vi "ControlSystemTemplate.vi"() -> ()   [LabVIEW 2012]
uses:
  SingleControls/TypeDef_LoopStages.ctl
  GlobalVariables_DIALMain.vi
  <vilib>/Utility/miscctls.llb/LVRectTypeDef.ctl
  <vilib>/Utility/miscctls.llb/LVPointTypeDef.ctl
panel:
  out "Commands Executed":i32
  in  "Reset Plot Bounds":bool
  out "Local Loop Stage":T1=enum."Exit"
  out "Total Errors":i32
  out "Permission Level":T2(ring)
  out "Local Queue Response":string="Exit Idle Loop"
  in  "Replot":bool
  in  "User Comment":bool
  in  "Update Permissions":bool
  in  "Software Testing":bool
  in  "Commanded Abort":bool
  out "Waiting Commands":i32
  out "Local Queue Element":string="Exit"
  in  "Local Abort":bool=TRUE
  # "Place Hidden Variables Here"
  # "Place Controls Here"
  # "Panel width is 954\nPanel height is 700 as child\nPanel height is 783 as stand alone"
  # "Place Queue Housekeeping Here"
  # "Place Global Buttons Here"
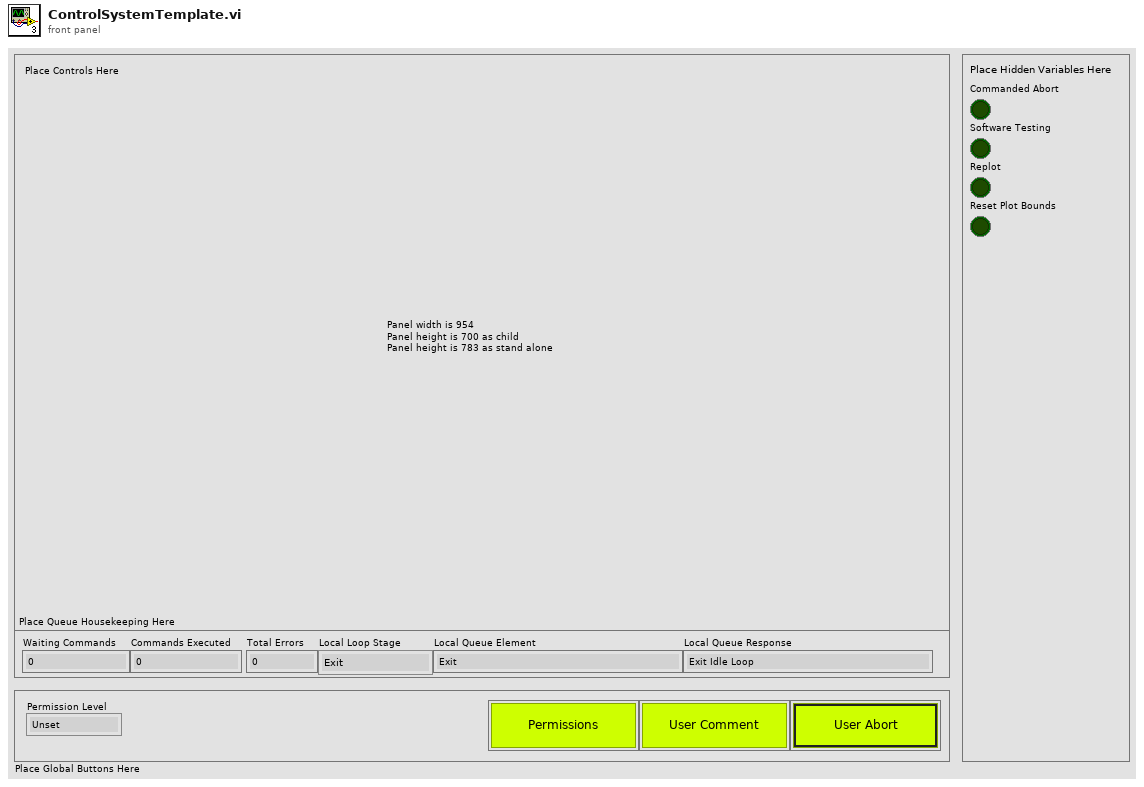
[diagram p1: front panel]
types:
  T1 = typedef "TypeDef_LoopStages.ctl" = enum16{"Configure", "Initialize", "Idle", "Error Handler", "Commanded Exit", "Exit"}
  T2 = enum16{"Unset", "Operator", "Administrator", "Full"}
  T3 = typedef "LVPointTypeDef.ctl" = cluster{"Horizontal":i16, "Vertical":i16}
  T4 = typedef "LVRectTypeDef.ctl" = cluster{"Left":i16, "Top":i16, "Right":i16, "Bottom":i16}
  T5 = enum16{"Always On", "Always Off", "Off While Running"}
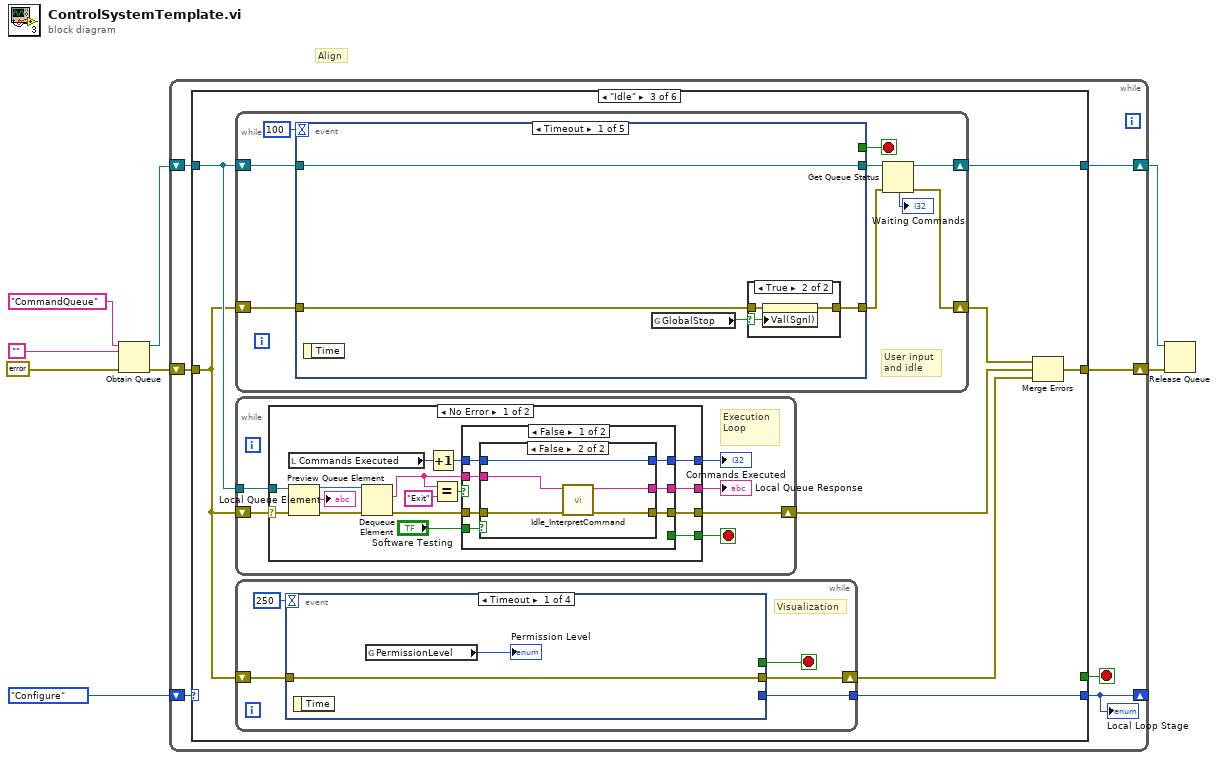
[diagram p0: block diagram]
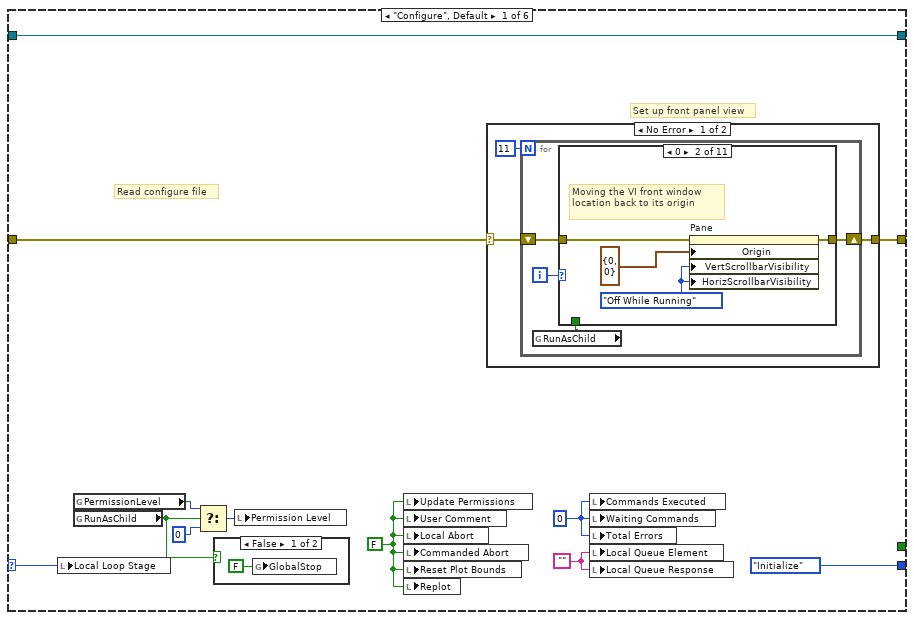
[diagram p2: hidden frame]
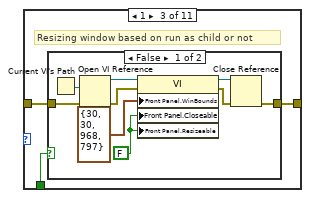
[diagram p5: hidden frame]
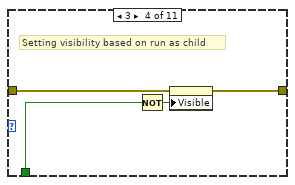
[diagram p7: hidden frame]
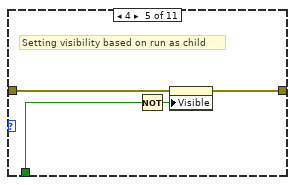
[diagram p8: hidden frame]
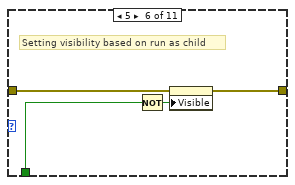
[diagram p9: hidden frame]
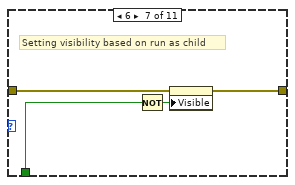
[diagram p10: hidden frame]
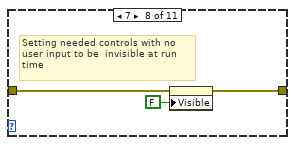
[diagram p11: hidden frame]
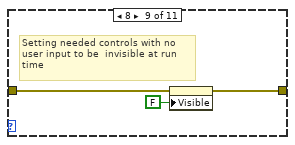
[diagram p12: hidden frame]
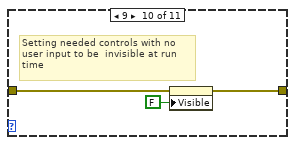
[diagram p13: hidden frame]
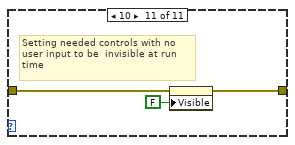
[diagram p14: hidden frame]
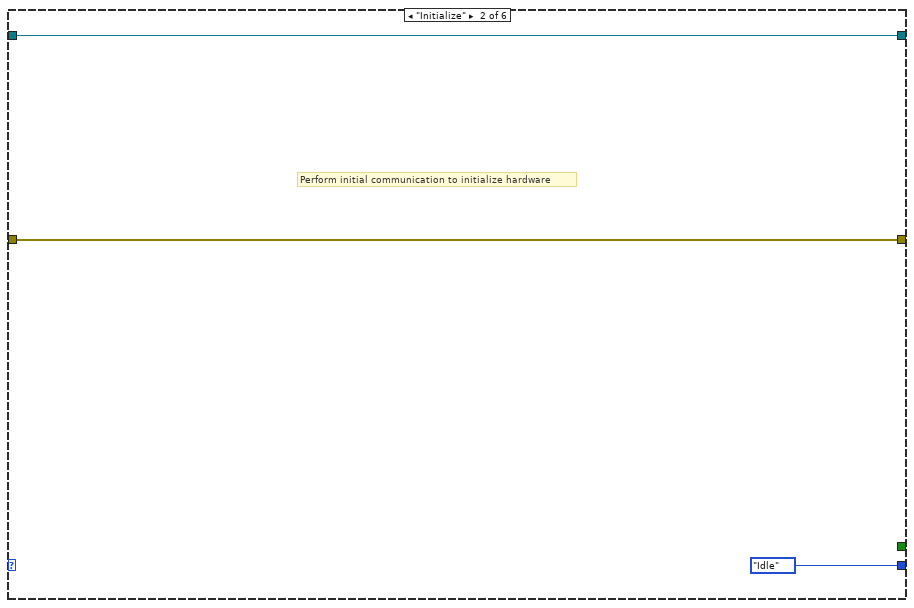
[diagram p16: hidden frame]
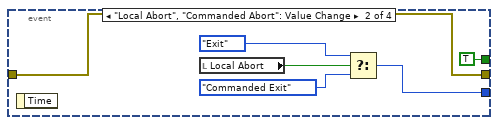
[diagram p17: hidden frame]
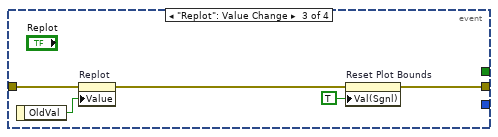
[diagram p18: hidden frame]
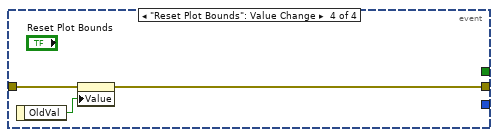
[diagram p19: hidden frame]
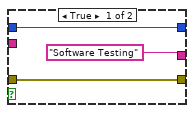
[diagram p20: hidden frame]
diagram:
  # "Align"
  n1 = Obtain Queue(name (unnamed)="CommandQueue", element data type="", error in (no error)=errorcluster {"status"=FALSE, "code"=0, "source"=""} ("error out")) -> (queue out=w3:refnum<queue>, error out=w1:errorcluster)  [unwired: 2 in, 1 out]
  n2 = while {
    shift-right: [w14] -> _
    shift-left: TypeDef_LoopStages."Configure" ("Enum") -> [w15]
    shift-right: [w12] -> w6
    shift-left: w1 -> [w10]
    shift-right: [w11] -> w7
    shift-left: w3 -> [w9]
    stop <- w13 stop-if-true
    n3 = case shown="\"Idle\"" w15 {
      selector: w15 -> [w26 _ _ _ _ _]
      tunnel: [TypeDef_LoopStages."Initialize" ("Enum") TypeDef_LoopStages."Idle" ("Enum") w86 TypeDef_LoopStages."Exit" ("Enum") TypeDef_LoopStages."Exit" ("Enum") TypeDef_LoopStages."Exit" ("Enum")] -> w14
      tunnel: [_ _ _ _ TRUE TRUE] -> w13
      tunnel: [w18 w84 w90 w200 w204 w207] -> w12
      tunnel: [w17 w83 w89 w201 w205 w209] -> w11
      tunnel: w10 -> [w20 w84 w88 w200 w204 w208]
      tunnel: w9 -> [w17 w83 w93 w201 w205 w209]
      frame "Configure", Default {
        w16 = 0 ("Waiting Commands")
        w24 = FALSE ("Local Abort")
        w25 = ""
        # "Read configure file"
        # "Set up front panel view"
        n4 = local write "Local Loop Stage"(w26) -> ()
        n5 = global read "GlobalVariables_DIALMain.vi" "PermissionLevel"() -> (w23:i32)
        n6 = global read "GlobalVariables_DIALMain.vi" "RunAsChild"() -> (w19:bool)
        n7 = Select(t=w23, s=w19, f=0) -> (s? t:f=w21:i32)
        n8 = case shown="False" w19 {
          frame False {
            n9 = global write "GlobalVariables_DIALMain.vi" "GlobalStop"(FALSE ("GlobalStop")) -> ()
          }
          frame True {
          }
        }
        n10 = local write "Permission Level"(w21) -> ()
        n11 = local write "Update Permissions"(w24) -> ()
        n12 = local write "User Comment"(w24) -> ()
        n13 = local write "Local Abort"(w24) -> ()
        n14 = local write "Commanded Abort"(w24) -> ()
        n15 = local write "Reset Plot Bounds"(w24) -> ()
        n16 = local write "Replot"(w24) -> ()
        n17 = case shown="No Error" w20 {
          selector: w20 -> [w31 w82]
          tunnel: [w30 w82] -> w18
          frame No Error {
            n18 = for {
              N: 11 -> [_]
              shift-right: [w33] -> w30
              shift-left: w31 -> [w34]
              i -> [w35]
              n19 = global read "GlobalVariables_DIALMain.vi" "RunAsChild"() -> (w32:bool)
              n20 = case shown="0" w35 {
                tunnel: w34 -> [w36 w39 w43 w55 w61 w64 w67 w71 w74 w77 w80]
                tunnel: [w36 w38 w42 w56 w60 w65 w68 w72 w75 w78 w81] -> w33
                tunnel: w32 -> [_ _ w41 w57 w58 w62 w69 _ _ _ _]
                frame -1, Default {
                }
                frame 0 {
                  w37 = T5."Off While Running" ("Vertical Scrollbar Visibility")
                  # "Moving the VI front window location back to its origin"
                  n21 = property on="Pane" class="Pane"(error in=w39, "Origin"=T3 {"Horizontal"=0, "Vertical"=0}, "VertScrollbarVisibility"=w37, "HorizScrollbarVisibility"=w37) -> (error out=w38:errorcluster)  [unwired: 1 in, 1 out]
                }
                frame 1 {
                  # "Resizing window based on run as child or not"
                  n22 = case shown="False" w41 {
                    tunnel: w43 -> [w51 w53]
                    tunnel: [w46 w53] -> w42
                    frame False {
                      w44 = FALSE
                      n23 = Current VI's Path() -> (path=w52:path)
                      n24 = Open VI Reference(vi path=w52, error in (no error)=w51) -> (vi reference=w50:refnum<vi>, error out=w49:errorcluster)  [unwired: 4 in]
                      n25 = property class="VI"(reference=w50, error in=w49, "Front Panel.WinBounds"=T4 {"Left"=30, "Top"=30, "Right"=968, "Bottom"=797} ("Front Panel Window:Panel Bounds"), "Front Panel.Closeable"=w44, "Front Panel.Resizeable"=w44) -> (reference out=w48:refnum<vi>, error out=w47:errorcluster)
                      n26 = Close Reference(reference=w48, error in (no error)=w47) -> (error out=w46:errorcluster)
                    }
                    frame True {
                    }
                  }
                }
                frame 3 {
                  # "Setting visibility based on run as child"
                  n27 = Not(x=w57) -> (.not. x?=w54:bool)
                  n28 = property on="Permission Level" class="Enum (strict)"(error in=w55, "Visible"=w54) -> (error out=w56:errorcluster)  [unwired: 1 in, 1 out]
                }
                frame 4 {
                  # "Setting visibility based on run as child"
                  n29 = Not(x=w58) -> (.not. x?=w59:bool)
                  n30 = property on="Update Permissions" class="Bool (strict)"(error in=w61, "Visible"=w59) -> (error out=w60:errorcluster)  [unwired: 1 in, 1 out]
                }
                frame 5 {
                  # "Setting visibility based on run as child"
                  n31 = Not(x=w62) -> (.not. x?=w63:bool)
                  n32 = property on="User Comment" class="Bool (strict)"(error in=w64, "Visible"=w63) -> (error out=w65:errorcluster)  [unwired: 1 in, 1 out]
                }
                frame 6 {
                  # "Setting visibility based on run as child"
                  n33 = Not(x=w69) -> (.not. x?=w66:bool)
                  n34 = property on="Local Abort" class="Bool (strict)"(error in=w67, "Visible"=w66) -> (error out=w68:errorcluster)  [unwired: 1 in, 1 out]
                }
                frame 7 {
                  # "Setting needed controls with no user input to be  invisible at run time"
                  n35 = property on="Commanded Abort" class="Bool (strict)"(error in=w71, "Visible"=FALSE) -> (error out=w72:errorcluster)  [unwired: 1 in, 1 out]
                }
                frame 8 {
                  # "Setting needed controls with no user input to be  invisible at run time"
                  n36 = property on="Software Testing" class="Bool (strict)"(error in=w74, "Visible"=FALSE) -> (error out=w75:errorcluster)  [unwired: 1 in, 1 out]
                }
                frame 9 {
                  # "Setting needed controls with no user input to be  invisible at run time"
                  n37 = property on="Replot" class="Bool (strict)"(error in=w77, "Visible"=FALSE) -> (error out=w78:errorcluster)  [unwired: 1 in, 1 out]
                }
                frame 10 {
                  # "Setting needed controls with no user input to be  invisible at run time"
                  n38 = property on="Reset Plot Bounds" class="Bool (strict)"(error in=w80, "Visible"=FALSE) -> (error out=w81:errorcluster)  [unwired: 1 in, 1 out]
                }
              }
            }
          }
          frame Error {
            # "Kill program because configuration failed"
          }
        }
        n39 = local write "Commands Executed"(w16) -> ()
        n40 = local write "Waiting Commands"(w16) -> ()
        n41 = local write "Total Errors"(w16) -> ()
        n42 = local write "Local Queue Element"(w25) -> ()
        n43 = local write "Local Queue Response"(w25) -> ()
      }
      frame "Initialize" {
        # "Perform initial communication to initialize hardware"
      }
      frame "Idle" {
        n44 = while {
          shift-right: [w164] -> w89
          shift-left: w93 -> [w168]
          shift-right: [w162] -> w92
          shift-left: w88 -> [w167]
          stop <- w166 stop-if-true
          # "User input\nand idle"
          n45 = event shown="[0] Timeout" {
            selector: _ -> [_ _ _ _ _]
            dyn-events: _ -> [_ _ _ _ _]
            timeout: 100 -> [_ _ _ _ _]
            tunnel: w168 -> [w173 w183 w185 w194 w199]
            tunnel: [w173 w179 w186 w190 w195] -> w165
            tunnel: w167 -> [w171 w181 w188 w192 w197]
            tunnel: [w170 w180 w187 w191 w196] -> w163
            tunnel: [_ TRUE ("LocalAbort") TRUE ("LocalAbort") _ _] -> w166
            event Timeout {
              n46 = event-data() -> ()  [unwired: 1 in, 1 out]
              n47 = global read "GlobalVariables_DIALMain.vi" "GlobalStop"() -> (w172:bool)
              n48 = case shown="True" w172 {
                selector: w172 -> [_ w175]
                tunnel: w171 -> [w174 w177]
                tunnel: [w174 w176] -> w170
                frame False {
                }
                frame True {
                  n49 = property on="Commanded Abort" class="Bool (strict)"(error in=w177, "Val(Sgnl)"=w175) -> (error out=w176:errorcluster)  [unwired: 1 in, 1 out]
                }
              }
            }
            event "Local Abort": Value Change {
              n50 = event-data() -> ()  [unwired: 1 in, 1 out]
              n51 = Enqueue Element At Opposite End(queue=w183, element="Exit", error in (no error)=w181) -> (queue out=w179:refnum<queue>, error out=w180:errorcluster)  [unwired: 1 in, 1 out]
            }
            event "Commanded Abort": Value Change {
              n52 = event-data() -> ()  [unwired: 1 in, 1 out]
              n53 = Enqueue Element At Opposite End(queue=w185, element="Exit", error in (no error)=w188) -> (queue out=w186:refnum<queue>, error out=w187:errorcluster)  [unwired: 1 in, 1 out]
            }
            event "Update Permissions": Value Change {
              n54 = event-data() -> ()  [unwired: 1 in, 1 out]
              n55 = Enqueue Element(queue=w194, element="System_OpenPermissionsVI", error in (no error)=w192) -> (queue out=w190:refnum<queue>, error out=w191:errorcluster)  [unwired: 1 in, 1 out]
            }
            event "User Comment": Value Change {
              n56 = event-data() -> ()  [unwired: 1 in, 1 out]
              n57 = Enqueue Element(queue=w199, element="System_OpenUserCommentVI", error in (no error)=w197) -> (queue out=w195:refnum<queue>, error out=w196:errorcluster)  [unwired: 1 in, 1 out]
            }
          }
          n58 = Get Queue Status(queue=w165, error in (no error)=w163) -> (queue out=w164:refnum<queue>, error out=w162:errorcluster, # elements in queue=→"Waiting Commands":i32)  [unwired: 1 in, 5 out]
        }
        n59 = while {
          tunnel: w93 -> [w118]
          shift-right: [w119] -> w91
          shift-left: w88 -> [w117]
          stop <- w120 stop-if-true
          # "Execution Loop"
          n60 = case shown="No Error" w117 {
            selector: w117 -> [w128 w160]
            tunnel: [w134 _] -> w120
            tunnel: [w131 w160] -> w119
            tunnel: w118 -> [w130 _]
            tunnel: [w126 "Error Loop Entered"] -> w116
            tunnel: [w123 w156] -> w115
            frame No Error {
              n61 = local read "Commands Executed"() -> (w125:i32)
              n62 = Preview Queue Element(queue=w130, error in (no error)=w128) -> (queue out=w129:refnum<queue>, element=→"Local Queue Element":string, error out=w136:errorcluster)  [unwired: 1 in, 1 out]
              n63 = Dequeue Element(queue=w129, error in (no error)=w136) -> (element=w121:string, error out=w132:errorcluster)  [unwired: 1 in, 2 out]
              n64 = Increment(x=w125) -> (x+1=w124:i32)
              n65 = Equal?(x=w121, y="Exit" ("x")) -> (x = y?=w133:bool)
              n66 = case shown="False" w133 {
                tunnel: w132 -> [w142 w154]
                tunnel: [w141 w154] -> w131
                tunnel: "Software Testing" -> [w143 _]
                tunnel: [_ TRUE] -> w134
                tunnel: [w140 "Exit Idle Loop"] -> w126
                tunnel: w124 -> [w139 w152]
                tunnel: [w138 w152] -> w123
                tunnel: w121 -> [w137 _]
                frame False {
                  n67 = case shown="False" w143 {
                    tunnel: w142 -> [w146 w150]
                    tunnel: [w146 w149] -> w141
                    tunnel: ["Software Testing" w147] -> w140
                    tunnel: w139 -> [w144 w151]
                    tunnel: [w144 w151] -> w138
                    tunnel: w137 -> [_ w148]
                    frame True {
                    }
                    frame False {
                      n68 = call "Idle_InterpretCommand.vi"("error in"=w150, "Input Command"=w148) -> ("error out"=w149:errorcluster, "What to Do"=w147:string)  [unwired: 8 in]
                    }
                  }
                }
                frame True {
                }
              }
            }
            frame Error {
              n69 = local read "Total Errors"() -> (w157:i32)
              n70 = Increment(x=w157) -> (x+1=→"Total Errors":i32)
              n71 = local read "Commands Executed"() -> (w156:i32)
            }
          }
          "Local Queue Response" <- w116
          "Commands Executed" <- w115
        }
        n72 = while {
          shift-right: [w96] -> w87
          shift-left: w88 -> [w97]
          tunnel: [w94] -> w86
          stop <- w95 stop-if-true
          # "Visualization"
          n73 = event shown="[0] Timeout" {
            selector: _ -> [_ _ _ _]
            dyn-events: _ -> [_ _ _ _]
            timeout: 250 -> [_ _ _ _]
            tunnel: w97 -> [w100 w105 w109 w114]
            tunnel: [w100 w105 w111 w113] -> w96
            tunnel: [_ TRUE ("LocalAbort") _ _] -> w95
            tunnel: [_ w101 _ _] -> w94
            event Timeout {
              n74 = event-data() -> ()  [unwired: 1 in, 1 out]
              n75 = global read "GlobalVariables_DIALMain.vi" "PermissionLevel"() -> (→"Permission Level":i32)
            }
            event "Local Abort", "Commanded Abort": Value Change {
              n76 = event-data() -> ()  [unwired: 1 in, 1 out]
              n77 = local read "Local Abort"() -> (w104:bool)
              n78 = Select(t=TypeDef_LoopStages."Exit" ("Enum"), s=w104, f=TypeDef_LoopStages."Commanded Exit" ("Enum")) -> (s? t:f=w101:T1)
            }
            event "Replot": Value Change {
              n79 = event-data() -> ("OldVal"=w107:bool)  [unwired: 1 in]
              n80 = property on="Replot" class="Bool (strict)"(error in=w109, "Value"=w107) -> (error out=w108:errorcluster)  [unwired: 1 in, 1 out]
              n81 = property on="Reset Plot Bounds" class="Bool (strict)"(error in=w108, "Val(Sgnl)"=TRUE ("Value (Signaling)")) -> (error out=w111:errorcluster)  [unwired: 1 in, 1 out]
            }
            event "Reset Plot Bounds": Value Change {
              n82 = event-data() -> ("OldVal"=w112:bool)  [unwired: 1 in]
              n83 = property on="Reset Plot Bounds" class="Bool (strict)"(error in=w114, "Value"=w112) -> (error out=w113:errorcluster)  [unwired: 1 in, 1 out]
            }
          }
        }
        n84 = Merge Errors(w92, w91, w87) -> (w90:errorcluster)
      }
      frame "Error Handler" {
      }
      frame "Commanded Exit" {
      }
      frame "Exit" {
        n85 = case shown="No Error" w208 {
          selector: w208 -> [w214 w244]
          tunnel: [w213 w244] -> w207
          frame No Error {
            n86 = for {
              N: 8 -> [_]
              shift-right: [w216] -> w213
              shift-left: w214 -> [w217]
              i -> [w218]
              n87 = case shown="-1, Default" w218 {
                tunnel: w217 -> [w219 w221 w224 w227 w230 w233 w236 w239 w242]
                tunnel: [w219 w222 w225 w228 w231 w234 w237 w240 w243] -> w216
                tunnel: TRUE ("Visible") -> [_ w220 w223 w226 w229 w232 w235 w238 w241]
                frame -1, Default {
                }
                frame 0 {
                  n88 = property on="Permission Level" class="Enum (strict)"(error in=w221, "Visible"=w220) -> (error out=w222:errorcluster)  [unwired: 1 in, 1 out]
                }
                frame 1 {
                  n89 = property on="Update Permissions" class="Bool (strict)"(error in=w224, "Visible"=w223) -> (error out=w225:errorcluster)  [unwired: 1 in, 1 out]
                }
                frame 2 {
                  n90 = property on="User Comment" class="Bool (strict)"(error in=w227, "Visible"=w226) -> (error out=w228:errorcluster)  [unwired: 1 in, 1 out]
                }
                frame 3 {
                  n91 = property on="Local Abort" class="Bool (strict)"(error in=w230, "Visible"=w229) -> (error out=w231:errorcluster)  [unwired: 1 in, 1 out]
                }
                frame 4 {
                  n92 = property on="Commanded Abort" class="Bool (strict)"(error in=w233, "Visible"=w232) -> (error out=w234:errorcluster)  [unwired: 1 in, 1 out]
                }
                frame 5 {
                  n93 = property on="Software Testing" class="Bool (strict)"(error in=w236, "Visible"=w235) -> (error out=w237:errorcluster)  [unwired: 1 in, 1 out]
                }
                frame 6 {
                  n94 = property on="Replot" class="Bool (strict)"(error in=w239, "Visible"=w238) -> (error out=w240:errorcluster)  [unwired: 1 in, 1 out]
                }
                frame 7 {
                  n95 = property on="Reset Plot Bounds" class="Bool (strict)"(error in=w242, "Visible"=w241) -> (error out=w243:errorcluster)  [unwired: 1 in, 1 out]
                }
              }
            }
          }
          frame Error {
          }
        }
      }
    }
    "Local Loop Stage" <- w14
  }
  n96 = Release Queue(queue=w7, error in (no error)=w6) -> ()  [unwired: 1 in, 3 out]
